vi "ADQ214 Set Sample Skip.vi"(8 "error in (no error)":errorcluster, 9 "skipfactor":u32, 10 "adq214_num":i32, 11 "adq_cu_ptr":u32) -> (0 "error out":errorcluster, 2 "function return":u32, 3 "adq_cu_ptr out":u32)   [LabVIEW 2013]
doc: "extern \"C\" __declspec(dllimport) unsigned int ADQ214_SetSampleSkip(void* adq_cu_ptr, int adq214_num, unsigned int skipfactor);"
uses:
  dlls/ADQAPI.dll
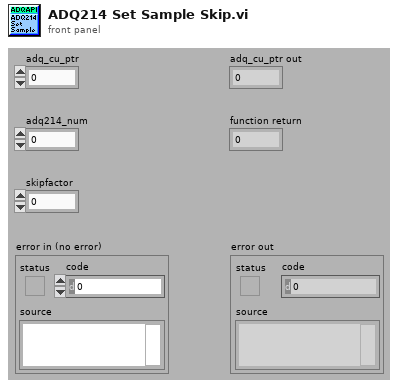
[diagram p1: front panel]
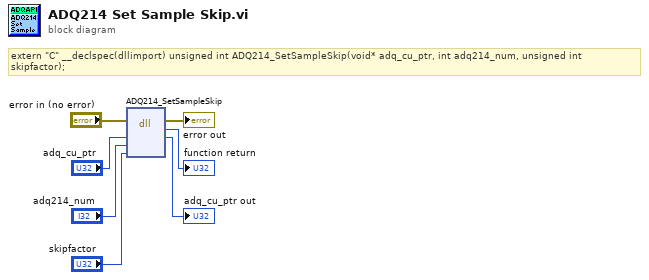
[diagram p0: block diagram]
diagram:
  # "extern \"C\" __declspec(dllimport) unsigned int\tADQ214_SetSampleSkip(void* adq_cu_ptr, int adq214_num, unsigned int skipfactor);"
  n1 = dll-call lib="C:/Users/astafiev/Desktop/IlyaDrive/@photonCounting/LabView_Imperium/dlls/ADQAPI.*" fn="ADQ214_SetSampleSkip"(error in="error in (no error)", "adq_cu_ptr"="adq_cu_ptr", "adq214_num"="adq214_num", "skipfactor"="skipfactor") -> (error out=→"error out":errorcluster, "return type"=→"function return":u32, "adq_cu_ptr"=→"adq_cu_ptr out":u32)  [unwired: 4 in, 1 out]
